vi "TTL.vi"(11 "MV":dbl(slide) scale=-100.0..100.0) -> ()   [LabVIEW 2018]
panel:
  in  "stop":bool
  out "TTL":bool
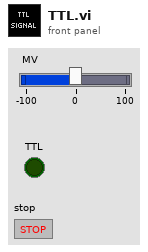
[diagram p1: front panel]
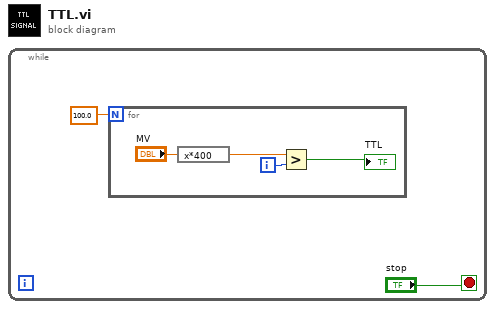
[diagram p0: block diagram]
diagram:
  n1 = while {
    stop <- "stop" stop-if-true
    n2 = for {
      N: 100.0 -> [_]
      i -> [w6]
      n3 = expression code="x*400"("MV") -> (w5:dbl)
      n4 = Greater?(x=w5, y=w6) -> (0:→"TTL":bool)
    }
  }
